vi "Resize FP.vi"(0 "VI in":refnum<vi>, 11 "error in":errorcluster) -> (4 "VI out":refnum<vi>, 15 "error out":errorcluster)   [LabVIEW 2014]
uses:
  <vilib>/Utility/miscctls.llb/LVRectTypeDef.ctl
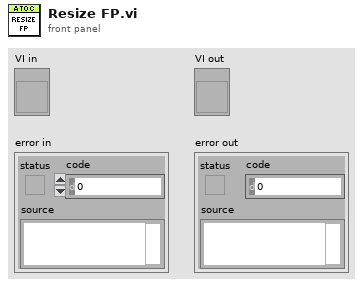
[diagram p1: front panel]
types:
  T1 = typedef "LVRectTypeDef.ctl" = cluster{"Left":i16, "Top":i16, "Right":i16, "Bottom":i16}
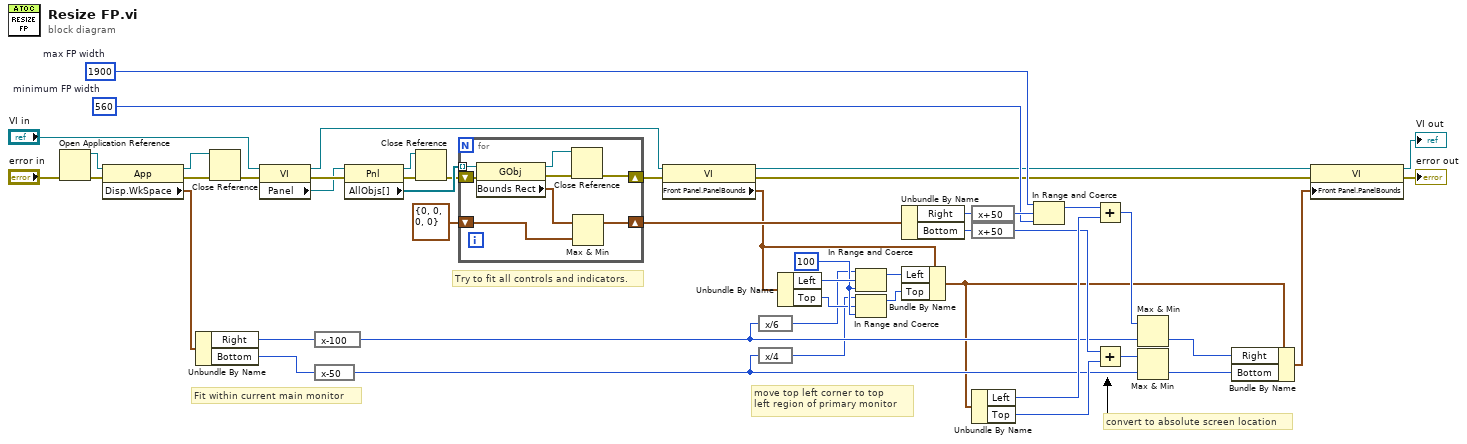
[diagram p0: block diagram]
diagram:
  w13 = i16 100 ("lower limit")
  w15 = i16 1900  # max FP width
  w16 = i16 560  # minimum FP width
  # "move top left corner to top\nleft region of primary monitor"
  # "convert to absolute screen location"
  # "Try to fit all controls and indicators."
  # "Fit within current main monitor"
  n1 = Open Application Reference(8:"error in") -> (0:w41:errorcluster, 3:w45:refnum<vi>)  [unwired: 3 in]
  n2 = property class="App"(reference=w45, error in=w41) -> (reference out=w43:refnum<vi>, error out=w42:errorcluster, "Disp.WkSpace"=w44:T1)
  n3 = Unbundle By Name(w44) -> ("Right"=w38:i16, "Bottom"=w37:i16)
  n4 = Close Reference(reference=w43, error in (no error)=w42) -> (error out=w39:errorcluster)
  n5 = property class="VI"(reference="VI in", error in=w39) -> (reference out=w27:refnum<vi>, error out=w33:errorcluster, "Panel"=w28:refnum<vi>)
  n6 = expression code="x-100"(w38) -> (w11:i16)
  n7 = expression code="x-50"(w37) -> (w10:i16)
  n8 = property class="Pnl"(reference=w28, error in=w33) -> (reference out=w30:refnum<vi>, error out=w32:errorcluster, "AllObjs[]"=w34:refnum<vi>[])
  n9 = Close Reference(reference=w30, error in (no error)=w32) -> (error out=w31:errorcluster)
  n10 = for {
    tunnel: w34 -> [w57] mode=indexing
    shift-right: [w54] -> w29
    shift-left: w31 -> [w56]
    shift-right: [w50] -> w25
    shift-left: T1 {"Left"=0, "Top"=0, "Right"=0, "Bottom"=0} ("Bounds Rect") -> [w51]
    n11 = property class="GObj"(reference=w57, error in=w56) -> (reference out=w53:refnum<vi>, error out=w55:errorcluster, "Bounds Rect"=w52:T1)
    n12 = Close Reference(reference=w53, error in (no error)=w55) -> (error out=w54:errorcluster)
    n13 = Max & Min(x=w52, y=w51) -> (max(x,y)=w50:T1)  [unwired: 1 out]
  }
  n14 = property class="VI"(reference=w27, error in=w29) -> (reference out=w7:refnum<vi>, error out=w6:errorcluster, "Front Panel.PanelBounds"=w2:T1)
  n15 = expression code="x/6"(w11) -> (w9:i16)
  n16 = expression code="x/4"(w10) -> (w8:i16)
  n17 = Unbundle By Name(w2) -> ("Left"=w14:i16, "Top"=w12:i16)
  n18 = In Range and Coerce(upper limit=w9, x=w14, lower limit=w13) -> (coerced(x)=w5:i16)  [unwired: 1 out]
  n19 = In Range and Coerce(upper limit=w8, x=w12, lower limit=w13) -> (coerced(x)=w4:i16)  [unwired: 1 out]
  n20 = Unbundle By Name(w25) -> ("Right"=w24:i16, "Bottom"=w23:i16)
  n21 = Bundle By Name(cluster=w2, "Left"=w5, "Top"=w4) -> (w3:T1)
  n22 = expression code="x+50"(w24) -> (w17:i16)
  n23 = expression code="x+50"(w23) -> (w36:i16)
  n24 = Unbundle By Name(w3) -> ("Left"=w46:i16, "Top"=w35:i16)
  n25 = In Range and Coerce(upper limit=w15, x=w17, lower limit=w16) -> (coerced(x)=w18:i16)  [unwired: 1 out]
  n26 = Add(x=w18, y=w46) -> (x+y=w22:i16)
  n27 = Add(x=w36, y=w35) -> (x+y=w21:i16)
  n28 = Max & Min(x=w22, y=w11) -> (min(x,y)=w20:i16)  [unwired: 1 out]
  n29 = Max & Min(x=w21, y=w10) -> (min(x,y)=w19:i16)  [unwired: 1 out]
  n30 = Bundle By Name(cluster=w3, "Right"=w20, "Bottom"=w19) -> (w1:T1)
  n31 = property class="VI"(reference=w7, error in=w6, "Front Panel.PanelBounds"=w1) -> (reference out=→"VI out":refnum<vi>, error out=→"error out":errorcluster)
